vi "Steering Controller.vi"(0 "Outer Loop State in":T1 {"Phi Setpoint" format="%#_13g"}, 7 "Steering On/off":bool, 9 "Inner Loop State in":T2, 11 "error in":errorcluster, 12 "PID Gains in":T3) -> (10 "Inner Loop State out":T2, 15 "error out":errorcluster)   [LabVIEW 2014]
uses:
  <vilib>/addons/control/pid/pid.llb/PID Structure.ctl
  <vilib>/addons/control/pid/pid.llb/PID Structure Conversion (DBL).vi
  <vilib>/addons/control/pid/pid.llb/PID (DBL).vi
  <userlib>/UCSD Robotics Lab/Robotics-Cape/LV/libroboticscape.lvlib
  <vilib>/addons/control/pid/NI_PID_pid.lvlib
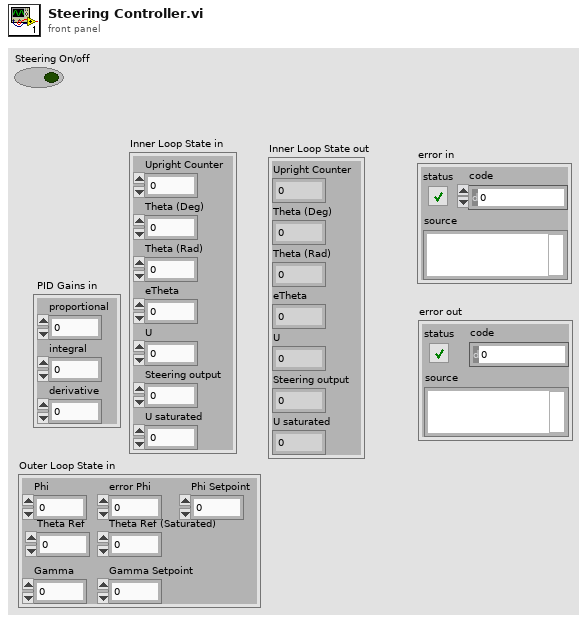
[diagram p1: front panel]
types:
  T1 = cluster{"Phi":dbl, "error Phi":dbl, "Gamma":dbl, "Theta Ref":dbl, "Theta Ref (Saturated)":sgl, "Gamma Setpoint":dbl, "Phi Setpoint":dbl}
  T2 = cluster{"Upright Counter":dbl, "Theta (Deg)":dbl, "Theta (Rad)":dbl, "eTheta":dbl, "U":dbl, "Steering output":dbl, "U saturated":sgl}
  T3 = cluster{"proportional":dbl, "integral":dbl, "derivative":dbl}
  T4 = typedef "NI_PID_pid.lvlib/PID Structure.ctl" = u16
  T5 = cluster{"proportional gain (Kc)":dbl, "integral time (Ti, min)":dbl, "derivative time (Td, min)":dbl}
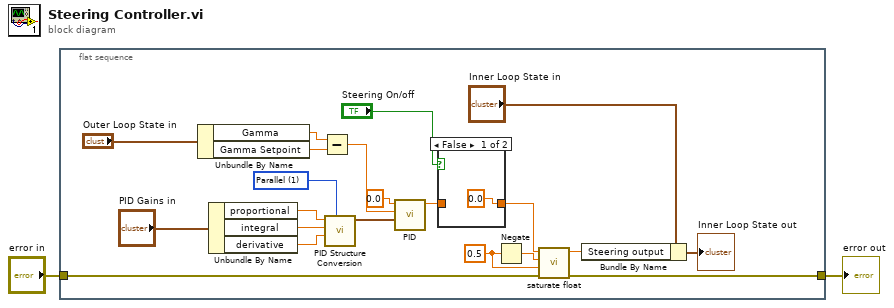
[diagram p0: block diagram]
diagram:
  n1 = flat-sequence {
    tunnel: "error in" -> [w15]
    tunnel: [w14] -> w1
    frame #0 {
      w23 = T4 1 items=["Academic (Standard)", "Parallel", "Series"] ("PID structure")
      w19 = sgl 0.5 ("min")
      n2 = Unbundle By Name("Outer Loop State in") -> ("Gamma"=w9:dbl, "Gamma Setpoint"=w3:dbl)
      n3 = Unbundle By Name("PID Gains in") -> ("proportional"=w18:dbl, "integral"=w17:dbl, "derivative"=w16:dbl)
      n4 = Subtract(x=w9, y=w3) -> (x-y=w13:dbl)
      n5 = call-poly <vilib>:"PID Structure Conversion.vi"("PID structure"=w23, "derivative"=w16, "integral"=w17, "proportional"=w18) -> ("PID gains"=w22:T5)  [unwired: 7 in]
      n6 = call-poly <vilib>:"PID.vi"("PID gains"=w22, "process variable"=w13, "setpoint"=0.0) -> ("output"=w8:dbl)  [unwired: 7 in, 1 out]
      n7 = case shown="False" "Steering On/off" {
        tunnel: w8 -> [_ w25]
        tunnel: [0.0 ("output") w25] -> w7
        frame False {
        }
        frame True {
        }
      }
      n8 = Negate(x=w19) -> (-x=w20:sgl)
      n9 = call <userlib>:"saturate float.vi"("error in (no error)"=w15, "max"=w19, "min"=w20, "val"=w7) -> ("error out"=w14:errorcluster, "val out"=w11:sgl)  [unwired: 5 in, 1 out]
      n10 = Bundle By Name(cluster="Inner Loop State in", "Steering output"=w11) -> (→"Inner Loop State out":T2)
    }
  }
  "error out" <- w1
